vi "Read Path type.vi"(8 "error in (no error)":errorcluster, 11 "SettingsFile in":refnum<class "SettingsFile.lvclass">) -> (0 "error out":errorcluster, 2 "Path type":bool, 3 "SettingsFile out":refnum<class "SettingsFile.lvclass">)   [LabVIEW 2013, in "SettingsFile.lvlib" / "SettingsFile.lvclass"]
uses:
  SettingsFile.lvclass
  SettingsFile.lvclass/SettingsFile.ctl
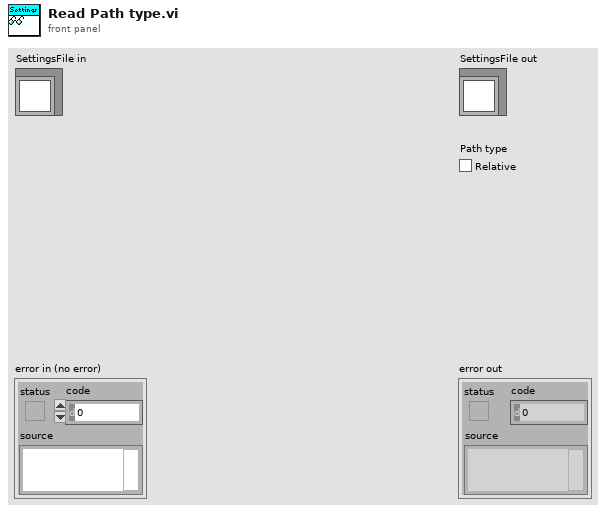
[diagram p1: front panel]
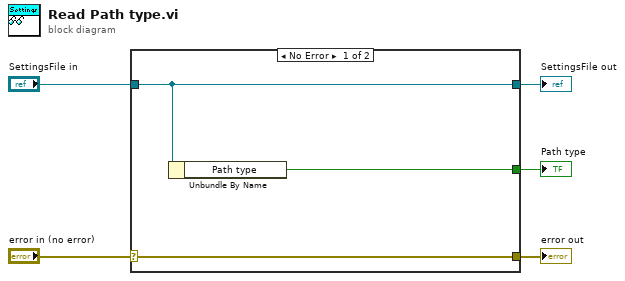
[diagram p0: block diagram]
diagram:
  n1 = case shown="No Error" "error in (no error)" {
    selector: "error in (no error)" -> [w8 w9]
    tunnel: [w8 w9] -> w4
    tunnel: [w7 w10] -> w2
    tunnel: "SettingsFile in" -> [w7 w10]
    tunnel: [w6 _] -> w1
    frame No Error {
      n2 = Unbundle By Name(w7) -> ("Path type"=w6:bool)
    }
    frame Error {
    }
  }
  "error out" <- w4
  "SettingsFile out" <- w2
  "Path type" <- w1
